vi "scanallchannels_test_calib.vi"(0 "Instrument VISA in":T1={"AWG VISA"="81160A", "Oscilloscope  VISA "="DSO80204B", "Integration Board IP"="172.16.7.43", "connection ID"=refnum, "report out"=refnum, "report file path"=path "D:/CTA/LevelTriggerBoardTest/TestsData/sumtrigger_delay"}, 2 "Save test data":bool=TRUE, 5 "Channels values":i32[](array[numeric])=[0, 1, 2, 3, 4, 5, 6], 7 "Channels init":i32[](array[numeric])=[1844, 1933, 1878, 1856, 2200, 1846, 1857], 9 "Cycles Burst":i32=10000, 11 "error in":errorcluster, 12 "L1 version":bool, 13 "Clipping":i32[][](array[numeric])) -> (4 "Instrument VISA out":T1={"AWG VISA"="81160A", "Oscilloscope  VISA "="DSO80204B", "Integration Board IP"="172.16.7.43", "connection ID"=refnum, "report out"=refnum, "report file path"=path "D:/CTA/LevelTriggerBoardTest/TestsData/sumtrigger_delay"}, 10 "Channels values":i32[](array[numeric])=[0, 1, 2, 3, 5, 6, 7], 15 "error out":errorcluster={"status"=TRUE, "code"=8, "source"=""})   [LabVIEW 2009]
doc: "This VI does a DTs calibration for Majority Trigger boards."
uses:
  <vilib>/Utility/NIReport.llb/NI_report.lvclass
  <vilib>/Utility/NIReport.llb/HTML/NI_HTML.lvclass
  <instrlib>/Agilent 81150/Agilent 81150.lvlib
panel:
  out "L1  50%":dbl[][][](array[numeric])
  out "x-y":i32[](array[numeric])=[-15, -75, -11, 0, -4, -22, -15]
  in  "Voltages values":dbl[](array[numeric])=[0.05, 0.1, 0.2, 0.3, 0.4, 0.5, 0.6, 0.7, 0.8, 0.9, 1.0, 1.1, 1.2, 1.3, 1.4, 1.5, 2.0, 2.5]
  out "report file path":path=path "D:/CTA/LevelTriggerBoardTest/TestsData/sumtrigger_delay"
  out "IPR_Address":i32=23
  out "L1 Address":i32=17
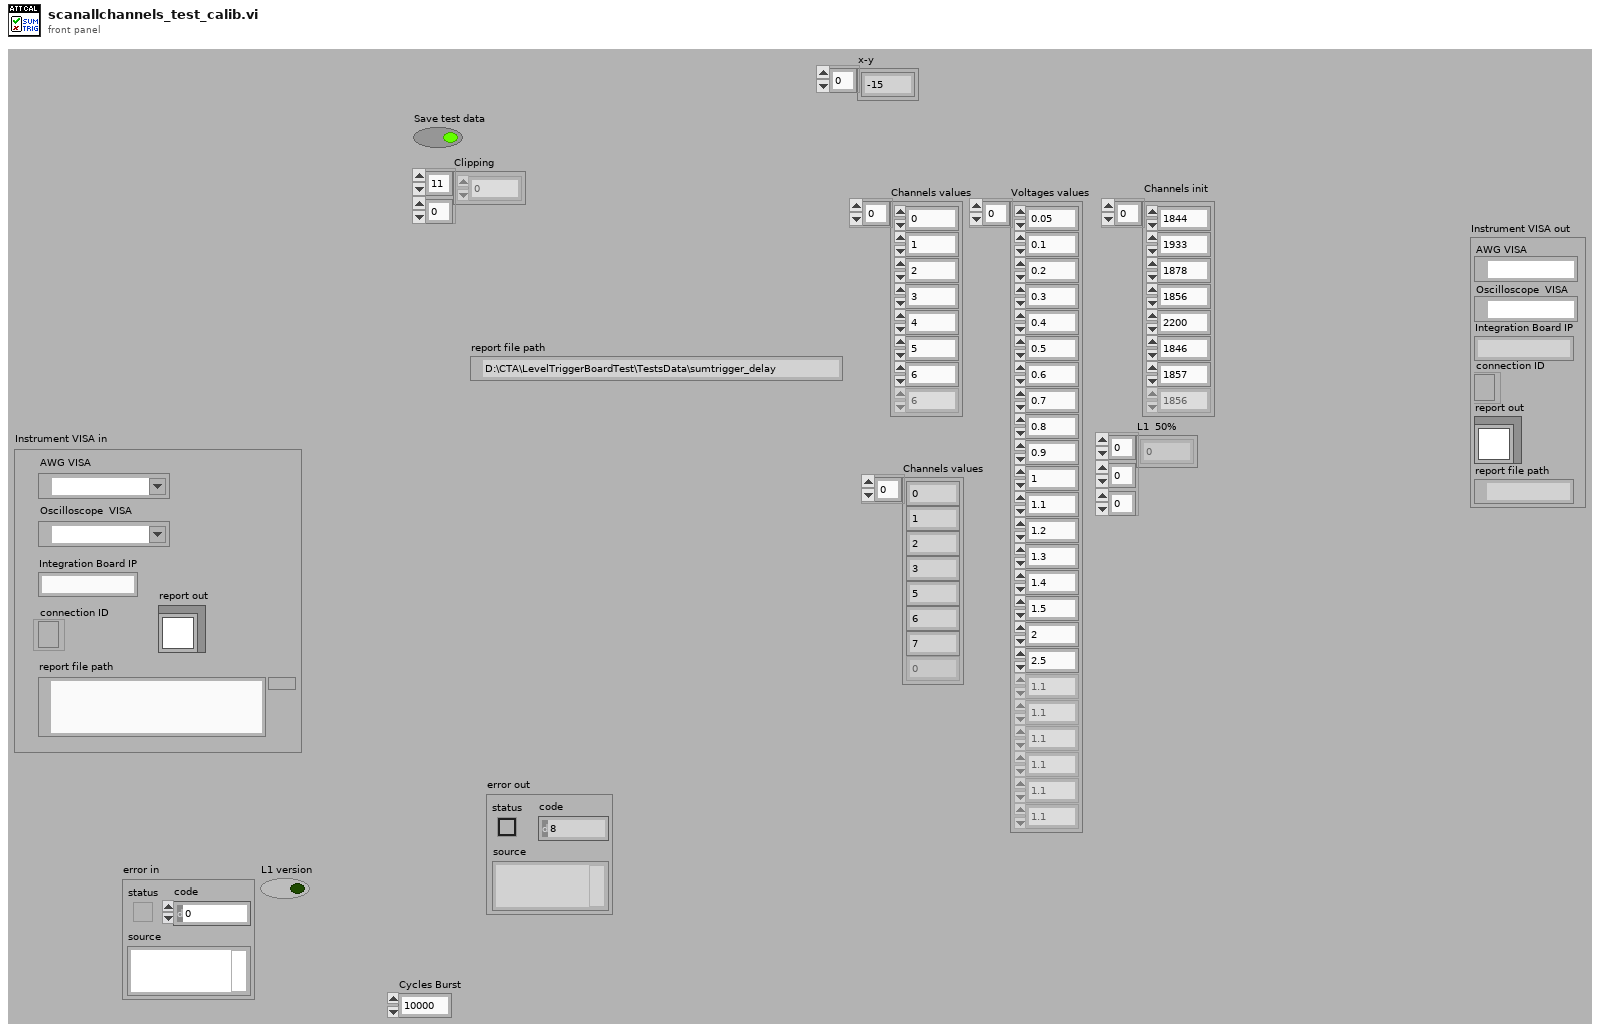
[diagram p1: front panel]
types:
  T1 = cluster{"AWG VISA":refnum<visa-resource-name>, "Oscilloscope  VISA ":refnum<visa-resource-name>, "Integration Board IP":string, "connection ID":refnum<k5>, "report out":refnum<class "NI_report.lvclass">, "report file path":path}
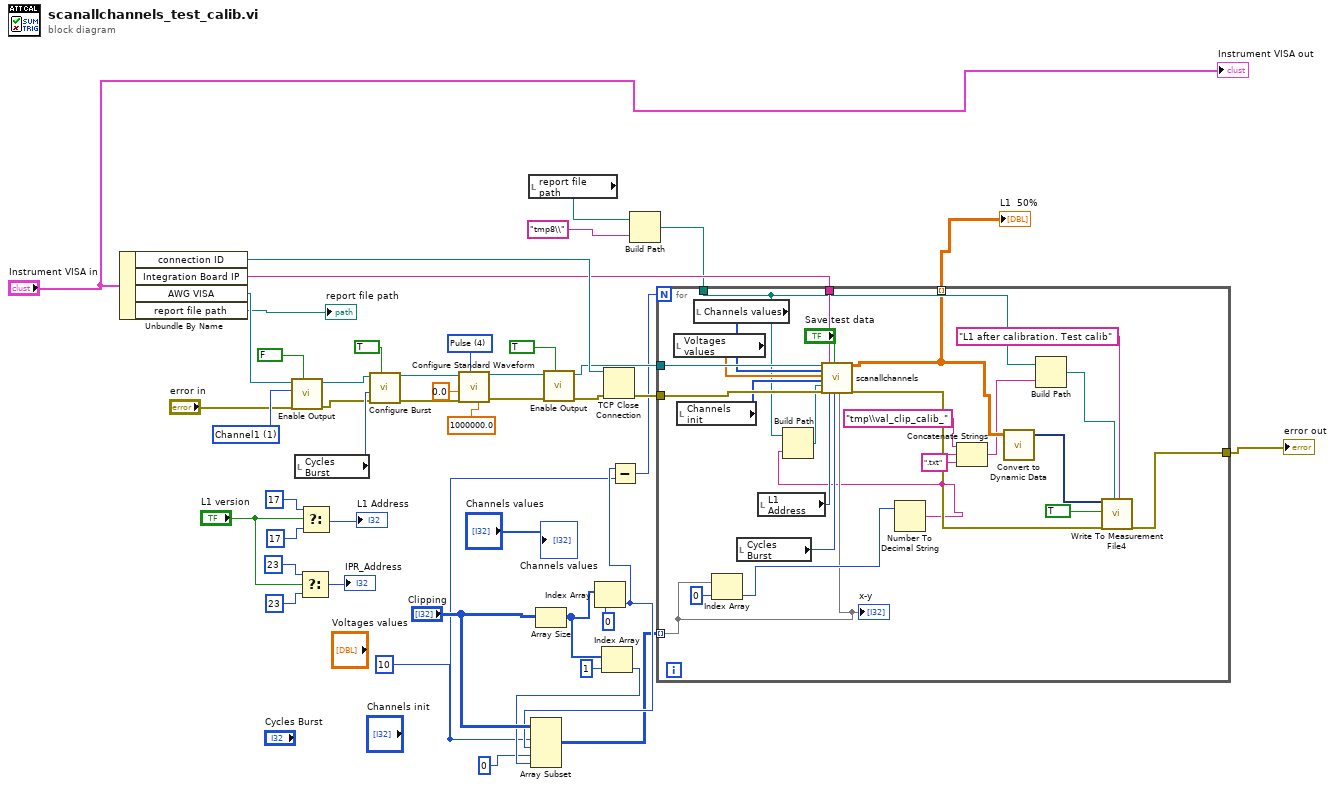
[diagram p0: block diagram]
diagram:
  w1 = 10 ("index")
  w38 = u16 4 items=["Sine", "Square", "Ramp Up", "Ramp Down", "Pulse", "Noise", "DC"] ("Waveform (0: Sine)")
  w45 = u16 1 items=["Channel1"=1, "Channel2"=2] ("Channel (1: Channel1)")
  n1 = Unbundle By Name("Instrument VISA in") -> ("connection ID"=w24:refnum<k5>, "Integration Board IP"=w16:string, "AWG VISA"=w39:refnum<visa-resource-name>, "report file path"=→"report file path":path)
  n2 = call <instrlib>:"Enable Output.vi"("Enable Output (T: Enable)"=FALSE, "error in (no error)"="error in", "Channel (1: Channel1)"=w45, "VISA resource name"=w39) -> ("error out"=w23:errorcluster, "VISA resource name out"=w22:refnum<visa-resource-name>)  [unwired: 6 in]
  n3 = local read "Cycles Burst"() -> (w26:i32)
  n4 = Select(t=23 ("Address"), s="L1 version", f=23 ("Address")) -> (s? t:f=→"IPR_Address":i32)
  n5 = Select(t=17 ("Address"), s="L1 version", f=17 ("Address")) -> (s? t:f=→"L1 Address":i32)
  n6 = call <instrlib>:"Configure Burst.vi"("Enable Burst (F: Disable)"=TRUE, "error in (no error)"=w23, "Burst Count (2)"=w26, "VISA resource name"=w22) -> ("error out"=w35:errorcluster, "VISA resource name out"=w36:refnum<visa-resource-name>)  [unwired: 6 in]
  n7 = call <instrlib>:"Configure Standard Waveform.vi"("Frequency (1000.0 Hz)"=1000000.0, "Waveform (0: Sine)"=w38, "error in (no error)"=w35, "Amplitude (1.0 Vpp)"=0.0, "VISA resource name"=w36) -> ("error out"=w34:errorcluster, "VISA resource name out"=w33:refnum<visa-resource-name>)  [unwired: 5 in]
  n8 = local read "report file path"() -> (w20:path)
  n9 = Array Size(array="Clipping") -> (size(s)=w8:i32[])
  n10 = call <instrlib>:"Enable Output.vi"("Enable Output (T: Enable)"=TRUE, "error in (no error)"=w34, "VISA resource name"=w33) -> ("error out"=w25:errorcluster, "VISA resource name out"=w17:refnum<visa-resource-name>)  [unwired: 7 in]
  n11 = Index Array(array=w8, index=0) -> (element=w4:i32)
  n12 = Index Array(array=w8, index=1) -> (element=w6:i32)
  n13 = Array Subset(array="Clipping", index (row)=w1, length (row)=w4, index (col)=0 ("index"), length (col)=w6) -> (w2:i32[][])
  n14 = TCP Close Connection(connection ID=w24, error in (no error)=w25) -> (error out=w18:errorcluster)  [unwired: 1 in, 1 out]
  n15 = Subtract(x=w4, y=w1) -> (x-y=w5:i32)
  n16 = Build Path(base path=w20, name or relative path="tmp8\\") -> (appended path=w13:path)
  n17 = for {
    N: w5 -> [_]
    tunnel: [w60] -> w12
    tunnel: w18 -> [w71]
    tunnel: w17 -> [w70]
    tunnel: w16 -> [w69]
    tunnel: w2 -> [w52] mode=indexing
    tunnel: w13 -> [w55]
    tunnel: [w54] -> w11 mode=indexing
    n18 = local read "Voltages values"() -> (w67:dbl[])
    n19 = local read "Channels init"() -> (w68:i32[])
    n20 = local read "Channels values"() -> (w66:i32[])
    n21 = Index Array(array=w52, index=0) -> (element=w56:i32)
    n22 = local read "Cycles Burst"() -> (w64:i32)
    n23 = local read "L1 Address"() -> (w65:i32)
    n24 = Number To Decimal String(number=w56) -> (decimal integer string=w50:string)  [unwired: 1 in]
    n25 = Build Path(base path=w55, name or relative path=w50) -> (appended path=w62:path)
    n26 = call "scanallchannels.vi"("VISA resource name out"=w70, "nm ch"=w66, "Voltages values"=w67, "Init ch value"=w68, "base path"=w62, "error in"=w71, "Integration Board IP"=w69, "L1 Address"=w65, "Save test data"="Save test data", "Ch burst"=w64, "vclip"=w52) -> ("L1  50%"=w54:dbl[][], "error out"=w61:errorcluster)  [unwired: 6 in, 1 out]
    n27 = Concatenate Strings("tmp\\val_clip_calib_" ("name or relative path"), w50, ".txt" ("string")) -> (w51:string)
    n28 = call "Convert to Dynamic Data"("2D Array"=w54) -> ("Dynamic Data Type"=w59:dynamicdata)  [unwired: 3 in]
    n29 = Build Path(base path=w55, name or relative path=w51) -> (appended path=w57:path)
    n30 = call "Write To Measurement File4"("Signals"=w59, "Enable"=TRUE, "error in (no error)"=w61, "Filename"=w57, "Comment"="L1 after calibration. Test calib") -> ("error out"=w60:errorcluster)  [unwired: 12 in, 2 out]
    "x-y" <- w52
  }
  "error out" <- w12
  "L1  50%" <- w11
  "Instrument VISA out" <- "Instrument VISA in"
  "Channels values" <- "Channels values"
